vi "Configure Chan Mode (Duty Cycle).vi"(4 "Chan DC Off (10)":i32=10, 6 "Chan DC On (10)":i32=10, 7 "Channel (1:Chan A)":i32(ring)=1 items=["Channel A"=1, "Channel B"=2, "Channel C"=3, "Channel D"=4, "Channel E"=5, "Channel F"=6, "Channel G"=7, "Channel H"=8], 8 "error in (no error)":errorcluster, 9 "Wait # (0)":i32, 11 "VISA resource name":refnum<visa-resource-name>) -> (0 "error out":errorcluster, 3 "VISA resource name out":refnum<visa-resource-name>)   [LabVIEW 2020, in "Berkeley Nucleonics 500 Series.lvlib"]
doc: "This VI is used to configure the duty cycle mode of operation for the selected channel."
uses:
  Berkeley Nucleonics 500 Series.lvlib
  Action-Status/Query Chan Parameters (Mode).vi
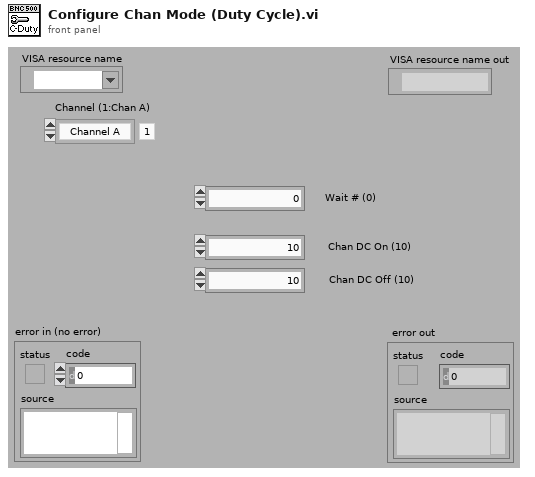
[diagram p1: front panel]
types:
  T1 = enum16{"Normal", "Single", "Burst", "Duty Cycle"}
  T2 = cluster{"Mode":enum16{"Normal", "Single", "Burst", "Duty Cycle"}, "Burst #":i32, "DC Off":i32, "DC On":i32, "Delay":dbl, "Width":dbl, "Wait #":i32}
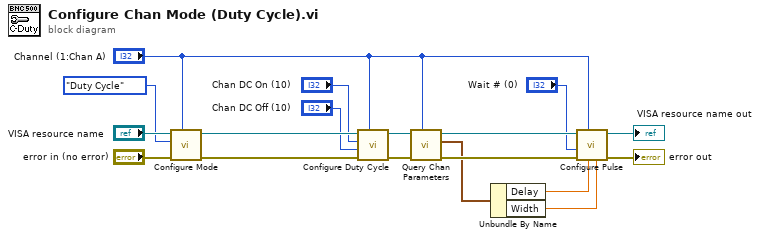
[diagram p0: block diagram]
diagram:
  n1 = call "Configure Mode.vi"("Channel (1:Chan A)"="Channel (1:Chan A)", "error in (no error)"="error in (no error)", "Mode (0:Normal)"=T1."Duty Cycle" ("Chan Mode"), "VISA resource name"="VISA resource name") -> ("error out"=w15:errorcluster, "VISA resource name out"=w16:refnum<visa-resource-name>)  [unwired: 6 in]
  n2 = call "Configure Duty Cycle.vi"("Channel (1:Chan A)"="Channel (1:Chan A)", "error in (no error)"=w15, "DC Off (10)"="Chan DC Off (10)", "DC On (10)"="Chan DC On (10)", "VISA resource name"=w16) -> ("error out"=w11:errorcluster, "VISA resource name out"=w10:refnum<visa-resource-name>)  [unwired: 5 in]
  n3 = call-poly "Query Chan Parameters.vi"("Channel (1: Chan A)"="Channel (1:Chan A)", "error in (no error)"=w11, "VISA resource name"=w10) -> ("error out"=w9:errorcluster, "Mode Parameters"=w4:T2, "VISA resource name out"=w8:refnum<visa-resource-name>)  [unwired: 6 in]
  n4 = Unbundle By Name(w4) -> ("Delay"=w2:dbl, "Width"=w1:dbl)
  n5 = call "Configure Pulse.vi"("Width (10 msec)"=w1, "Delay (10 msec)"=w2, "Channel (1:Chan A)"="Channel (1:Chan A)", "error in (no error)"=w9, "Wait # (0)"="Wait # (0)", "VISA resource name"=w8) -> ("error out"=→"error out":errorcluster, "VISA resource name out"=→"VISA resource name out":refnum<visa-resource-name>)  [unwired: 4 in]
